vi "Place Arrow Decoration.vi"(0 "Arrow Direction":T2, 1 "Diagram":refnum<vi>, 2 "Pane Refnum":refnum<vi>, 7 "FP? (T)":bool, 11 "error in":errorcluster, 12 "Pos":T1) -> (4 "Decor Refnum":refnum<vi>, 15 "error out":errorcluster)   [LabVIEW 2025]
uses:
  Arrow Direction.ctl
  <vilib>/Utility/miscctls.llb/LVPositionTypeDef.ctl
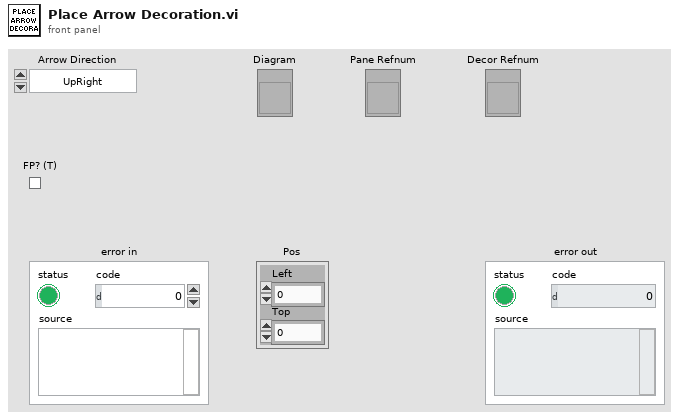
[diagram p1: front panel]
types:
  T1 = typedef "LVPositionTypeDef.ctl" = cluster{"Left":i32, "Top":i32}
  T2 = typedef "Arrow Direction.ctl" = enum16{"UpRight", "UpLeft", "DownLeft", "DownRight"}
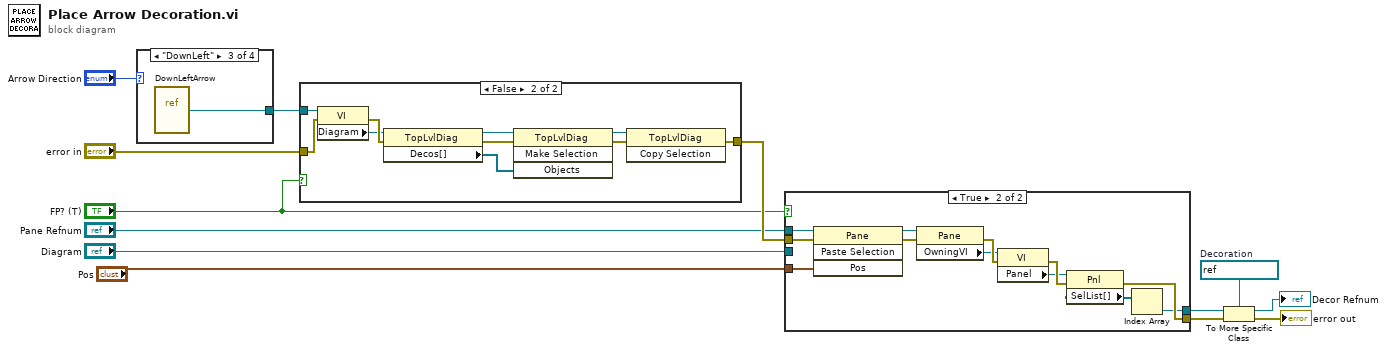
[diagram p0: block diagram]
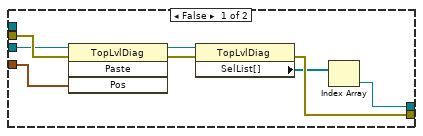
[diagram p2: hidden frame]
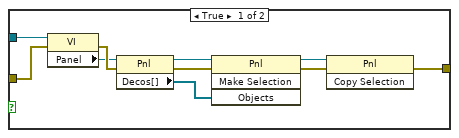
[diagram p3: hidden frame]
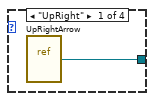
[diagram p4: hidden frame]
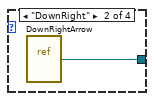
[diagram p5: hidden frame]
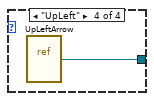
[diagram p6: hidden frame]
diagram:
  w4 = refnum<vi> refnum  # Decoration
  n1 = case shown="\"DownLeft\"" "Arrow Direction" {
    tunnel: [w14 w15 w16 w17] -> w9
    frame "UpRight" {
      n2 = vi-ref "UpRightArrow.vi"() -> (w14:refnum<vi>)
    }
    frame "DownRight" {
      n3 = vi-ref "DownRightArrow.vi"() -> (w15:refnum<vi>)
    }
    frame "DownLeft" {
      n4 = vi-ref "DownLeftArrow.vi"() -> (w16:refnum<vi>)
    }
    frame "UpLeft" {
      n5 = vi-ref "UpLeftArrow.vi"() -> (w17:refnum<vi>)
    }
  }
  n6 = case shown="False" "FP? (T)" {
    tunnel: w9 -> [w21 w31]
    tunnel: [w27 w36] -> w12
    tunnel: "error in" -> [w23 w33]
    frame True {
      n7 = property class="VI"(reference=w21, error in=w23) -> (error out=w24:errorcluster, "Panel"=w22:refnum<vi>)  [unwired: 1 out]
      n8 = property class="Pnl"(reference=w22, error in=w24) -> (reference out=w20:refnum<vi>, error out=w25:errorcluster, "Decos[]"=w19:refnum<vi>[])
      n9 = invoke class="Pnl" method="Make Selection"(reference=w20, error in=w25, "Objects"=w19) -> (reference out=w18:refnum<vi>, error out=w26:errorcluster)  [unwired: 1 in, 2 out]
      n10 = invoke class="Pnl" method="Copy Selection"(reference=w18, error in=w26) -> (error out=w27:errorcluster)  [unwired: 1 in, 2 out]
    }
    frame False {
      n11 = property class="VI"(reference=w31, error in=w33) -> (error out=w34:errorcluster, "Diagram"=w32:refnum<vi>)  [unwired: 1 out]
      n12 = property class="TopLvlDiag"(reference=w32, error in=w34) -> (reference out=w30:refnum<vi>, error out=w35:errorcluster, "Decos[]"=w29:refnum<vi>[])
      n13 = invoke class="TopLvlDiag" method="Make Selection"(reference=w30, error in=w35, "Objects"=w29) -> (reference out=w28:refnum<vi>, error out=w37:errorcluster)  [unwired: 1 in, 2 out]
      n14 = invoke class="TopLvlDiag" method="Copy Selection"(reference=w28, error in=w37) -> (error out=w36:errorcluster)  [unwired: 1 in, 2 out]
    }
  }
  n15 = case shown="True" "FP? (T)" {
    tunnel: w12 -> [w44 w57]
    tunnel: "Pane Refnum" -> [_ w51]
    tunnel: "Diagram" -> [w40 _]
    tunnel: [w39 w47] -> w6
    tunnel: [w43 w53] -> w11
    tunnel: "Pos" -> [w38 w46]
    frame False {
      n16 = invoke class="TopLvlDiag" method="Paste"(reference=w40, error in=w44, "Pos"=w38) -> (reference out=w42:refnum<vi>, error out=w45:errorcluster)  [unwired: 1 in, 2 out]
      n17 = property class="TopLvlDiag"(reference=w42, error in=w45) -> (error out=w43:errorcluster, "SelList[]"=w41:refnum<vi>[])  [unwired: 1 out]
      n18 = Index Array(array=w41) -> (element=w39:refnum<vi>)  [unwired: 1 in]
    }
    frame True {
      n19 = invoke class="Pane" method="Paste Selection"(reference=w51, error in=w57, "Pos"=w46) -> (reference out=w50:refnum<vi>, error out=w56:errorcluster)  [unwired: 1 in, 2 out]
      n20 = property class="Pane"(reference=w50, error in=w56) -> (error out=w55:errorcluster, "OwningVI"=w49:refnum<vi>)  [unwired: 1 out]
      n21 = property class="VI"(reference=w49, error in=w55) -> (error out=w54:errorcluster, "Panel"=w48:refnum<vi>)  [unwired: 1 out]
      n22 = property class="Pnl"(reference=w48, error in=w54) -> (error out=w53:errorcluster, "SelList[]"=w52:refnum<vi>[])  [unwired: 1 out]
      n23 = Index Array(array=w52) -> (element=w47:refnum<vi>)  [unwired: 1 in]
    }
  }
  n24 = To More Specific Class(target class=w4, reference=w6, error in=w11) -> (specific class reference=→"Decor Refnum":refnum<vi>, error out=→"error out":errorcluster)
